vi "convert rel chan num.vi"(8 "error in":errorcluster, 9 "Card":i32, 10 "Channel":i32, 11 "Crate":i32) -> (0 "error out":errorcluster, 1 "Crate index":i32, 2 "Absolute index":i32, 3 "ACTIVE index":i32)   [LabVIEW 2018]
uses:
  CAEN globals.vi
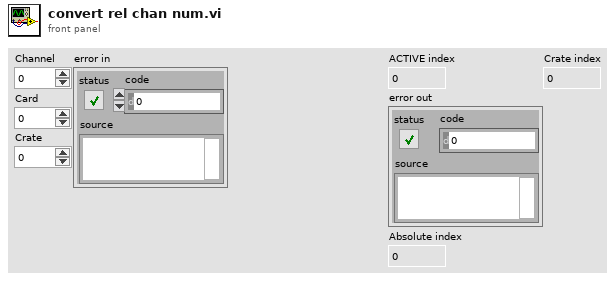
[diagram p1: front panel]
types:
  T1 = typedef "crate.ctl" = cluster{"CAENet Address":i32, "Crate Model":string, "Firmware Version":string, "Crate Map":T2[], "Total Channels":i32}
  T2 = typedef "card.ctl" = cluster{"Slot Number":i32, "Card Model":string, "Num Channels":i32, "Polarity":string, "Vmax":dbl, "Imax":dbl, "Revision":string}
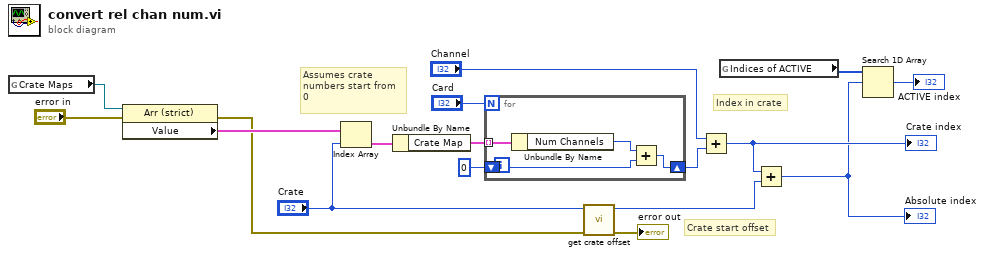
[diagram p0: block diagram]
diagram:
  # "Assumes crate \nnumbers start from\n0"
  # "Crate start offset"
  # "Index in crate"
  n1 = global read "CAEN globals.vi" "Crate Maps"() -> (w17:refnum<vi>)
  n2 = property class="Arr (strict)"(reference=w17, error in="error in") -> (error out=w2:errorcluster, "Value"=w8:T1[])  [unwired: 1 out]
  n3 = Index Array(array=w8, index="Crate") -> (element=w10:T1)
  n4 = Unbundle By Name(w10) -> ("Crate Map"=w15:T2[])
  n5 = for {
    N: "Card" -> [_]
    tunnel: w15 -> [w21] mode=indexing
    shift-right: [w18] -> w13
    shift-left: 0 -> [w19]
    n6 = Unbundle By Name(w21) -> ("Num Channels"=w20:i32)
    n7 = Add(x=w20, y=w19) -> (x+y=w18:i32)
  }
  n8 = call "get crate offset.vi"("error in"=w2, "Crate"="Crate") -> ("error out"=→"error out":errorcluster, "Start offset"=w4:i32)  [unwired: 8 in]
  n9 = Add(x="Channel", y=w13) -> (x+y=w9:i32)
  "Crate index" <- w9
  n10 = global read "CAEN globals.vi" "Indices of ACTIVE"() -> (w7:i32[])
  n11 = Add(x=w9, y=w4) -> (x+y=w6:i32)
  "Absolute index" <- w6
  n12 = Search 1D Array(1D array=w7, element=w6) -> (index of element=→"ACTIVE index":i32)  [unwired: 1 in]
